vi "ReadDriverParameters.vi"(8 "error in (no error)":errorcluster) -> (0 "error out":errorcluster, 2 "DRV stand":T1)   [LabVIEW 2018, in "Application.lvlib"]
doc: "Read Driver Parameters in an Excel file"
uses:
  Application/Application.lvlib
  Application/DRV stand.ctl
  <vilib>/Utility/NIReport.llb/Report Type.ctl
  <vilib>/addons/_office/excel.llb/Excel Get Data ([str]).vi
  <vilib>/Utility/NIReport.llb/NI_report.lvclass
  <vilib>/Utility/NIReport.llb/Excel/NI_Excel.lvclass
  <vilib>/addons/_office/NI_ReportGenerationToolkit.lvlib
  <vilib>/Utility/NIReport.llb/NI_ReportGenerationCore.lvlib
panel:
  in  "effeciency":bool
  in  "DCI":bool
  in  "DCV":bool=TRUE
  in  "kW":bool=TRUE
  in  "PF":bool=TRUE
  in  "ACI":bool=TRUE
  in  "ACV":bool=TRUE
  in  "Cancel":bool
  out "Name":string
  out "effect min":dbl caption="HIÖU SUÊT"
  out "effect max":dbl caption="HIÖU SUÊT"
  out "DCI(mA) min":dbl caption="§IÖN ¸P DC (mA)"
  out "DCI(mA) max":dbl caption="§IÖN ¸P DC (mA)"
  out "DCV(Volts) min":dbl caption="§IÖN ¸P DC (Volts)"
  out "DCV(Volts) max":dbl caption="§IÖN ¸P DC (Volts)"
  out "AC kW (W) min":dbl caption="C¤NG SUÊT AC (Watt)"
  out "AC kW (W) max":dbl caption="C¤NG SUÊT AC (Watt)"
  out "pf min":dbl caption="HÖ Sè C¤NG SUÊT"
  out "pf  max":dbl caption="HÖ Sè C¤NG SUÊT"
  out "ACI(mA) min":dbl caption="DßNG §IÖN AC (mA)"
  out "ACI(mA) max":dbl caption="DßNG §IÖN AC (mA)"
  out "ACV(Volts) min":dbl caption="§iÖn ¸p AC (Volts)"
  out "ACV(Volts) max":dbl caption="§iÖn ¸p AC (Volts)"
  in  "Select Excel File":bool
  in  "Select":bool
  in  "ID":u16(ring) items=["00037845", "00032982", "00035647", "00035625", "00029051", "00039782", "00039558", "00041093", "00039479", "00022963", "00027236", "00029031", "00040386", "00040388", "00040390", "00030784", "00040761", "00040392", "00040394", "00040396", "00039185", "00041068", "00041072", "00041471", "00041079", "00027769", "00018946", "00026890", "00023932", "00040779", "00026346", "00027544", "00028946", "00039696", "00023152", "00015630", "00034834", "00035257", "00035244", "00041789", "00027814", "00028354", "00032423", "00031816", "00041407", "00039539", "00039236"]
  out "Parameters":string[](array[string])
  # "DRIVER"
  # "Parameters"
  # "MAX"
  # "MIN"
  # "§IÖN ¸P AC (Volts)"
  # "Dßng §IÖn AC (mA)"
  # "HÖ sè c«ng suÊt"
  # "c«ng suÊt AC (Watt)"
  # "§IÖN ¸P DC (VOLTS)"
  # "DßNG §IÖN DC (mA)"
  # "HIÖU SUÊT"
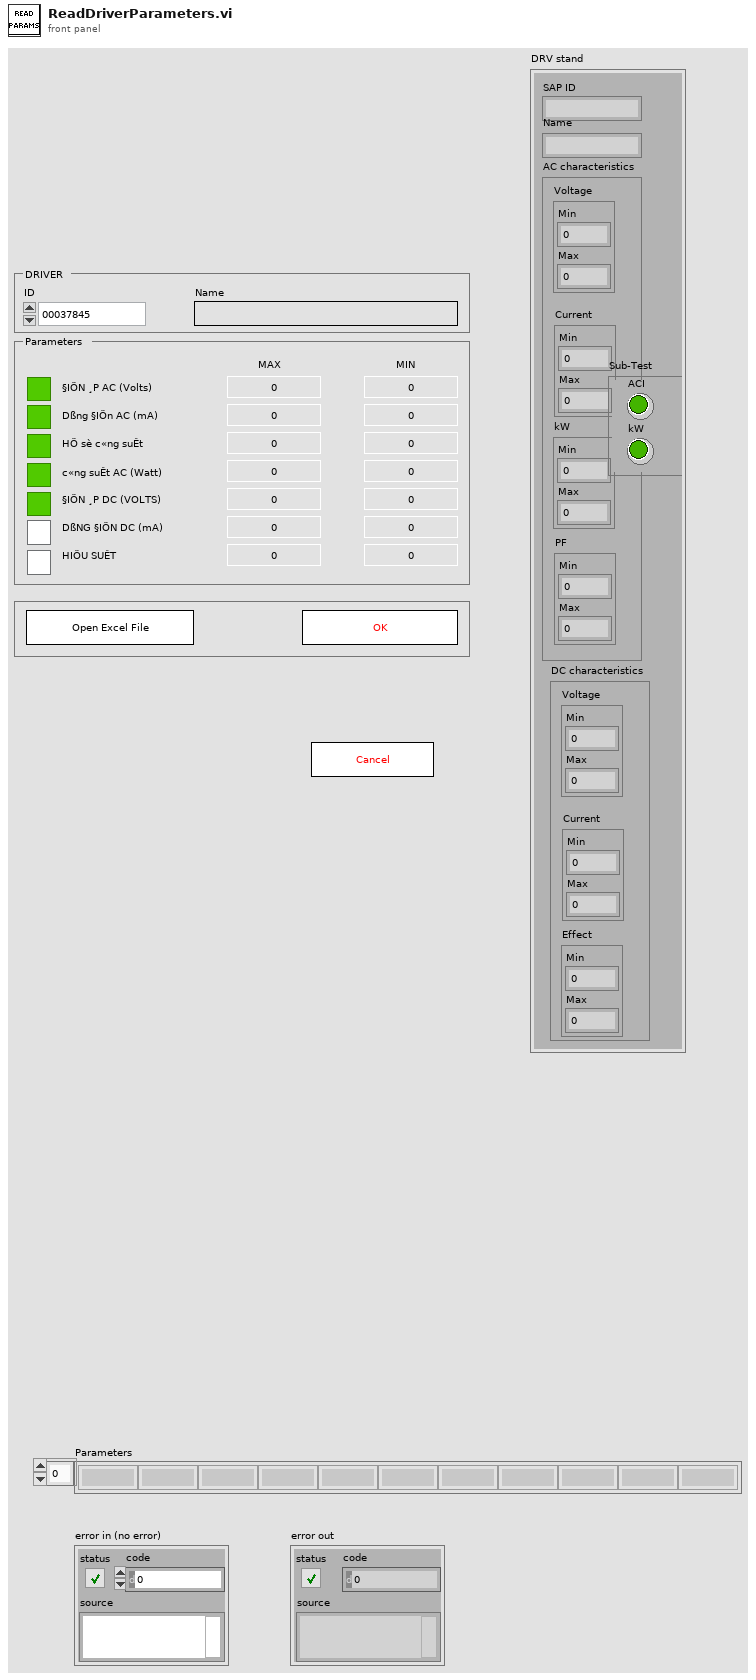
[diagram p1: front panel]
types:
  T1 = typedef "Application.lvlib/DRV stand.ctl" = cluster{"SAP ID":string, "Name":string, "AC characteristics":cluster{"Voltage":cluster{"Min":dbl, "Max":dbl}, "Current":cluster{"Min":dbl, "Max":dbl}, "kW":cluster{"Min":dbl, "Max":dbl}, "PF":cluster{"Min":dbl, "Max":dbl}}, "DC characteristics":cluster{"Voltage":cluster{"Min":dbl, "Max":dbl}, "Current":cluster{"Min":dbl, "Max":dbl}, "Effect":cluster{"Min":dbl, "Max":dbl}}, "Sub-Test":cluster{"ACV":bool, "ACI":bool, "kW":bool, "PF":bool, "DCV":bool, "DCI":bool, "efficiency":bool}}
  T2 = enum16{"maximized", "minimized", "normal", "no change"}
  T3 = typedef "NI_ReportGenerationCore.lvlib/Report Type.ctl" = enum16{"HTML", "Word", "Excel"}
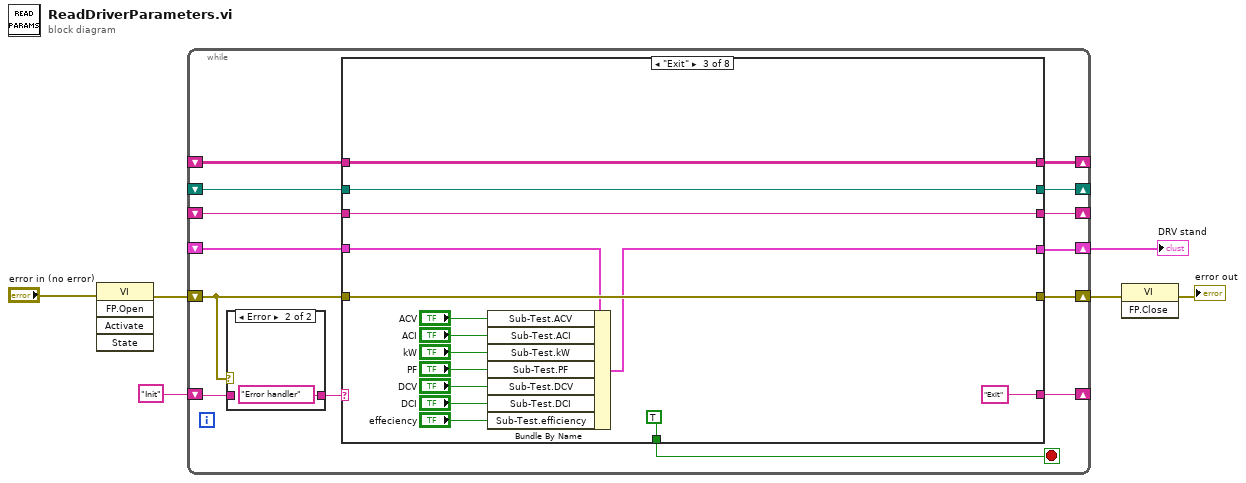
[diagram p0: block diagram]
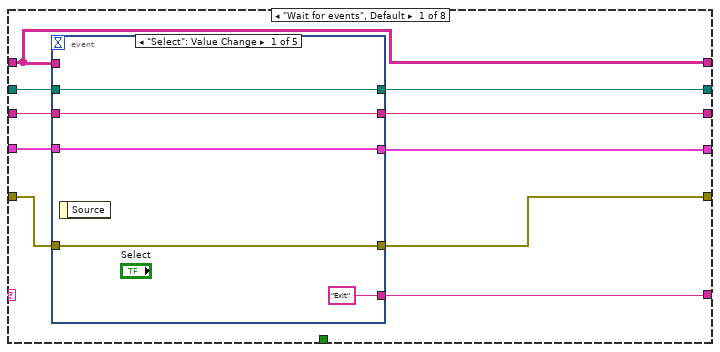
[diagram p3: hidden frame]
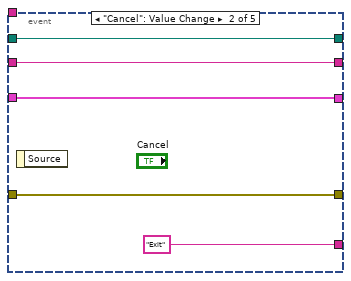
[diagram p4: hidden frame]
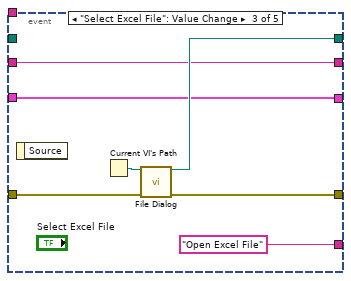
[diagram p5: hidden frame]
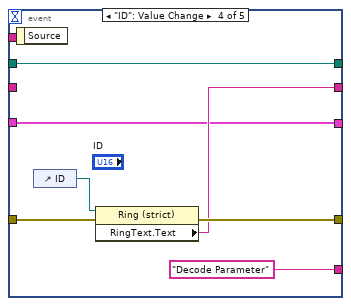
[diagram p6: hidden frame]
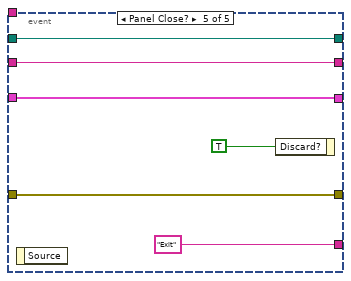
[diagram p7: hidden frame]
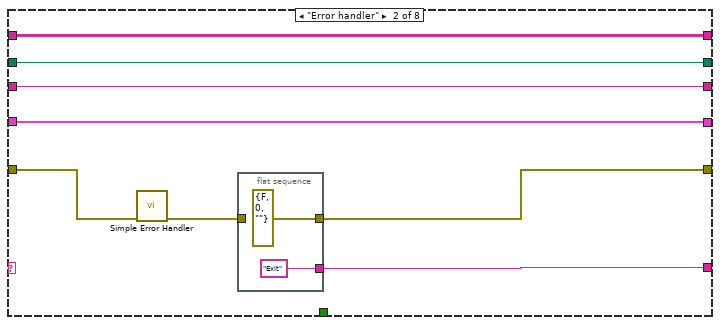
[diagram p8: hidden frame]
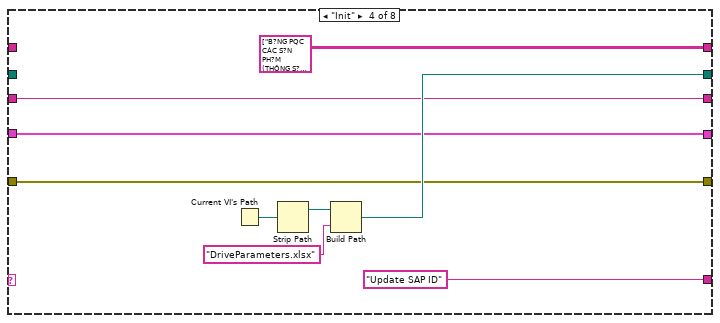
[diagram p9: hidden frame]
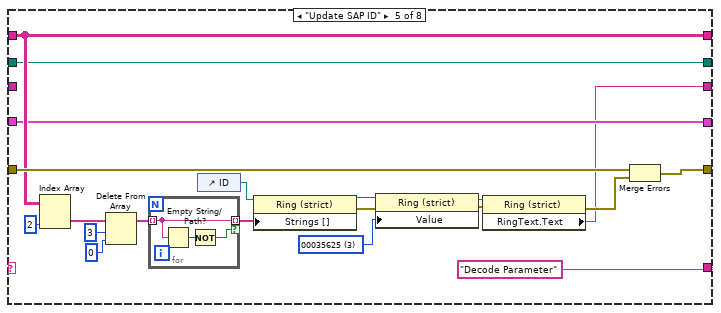
[diagram p10: hidden frame]
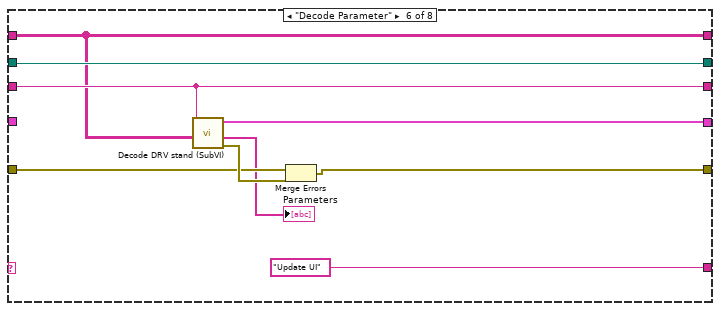
[diagram p11: hidden frame]
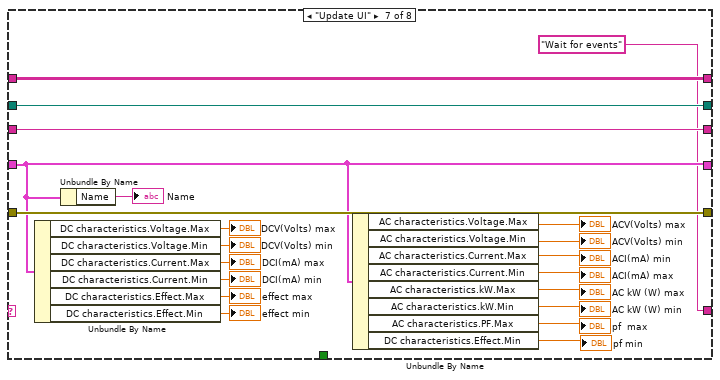
[diagram p12: hidden frame]
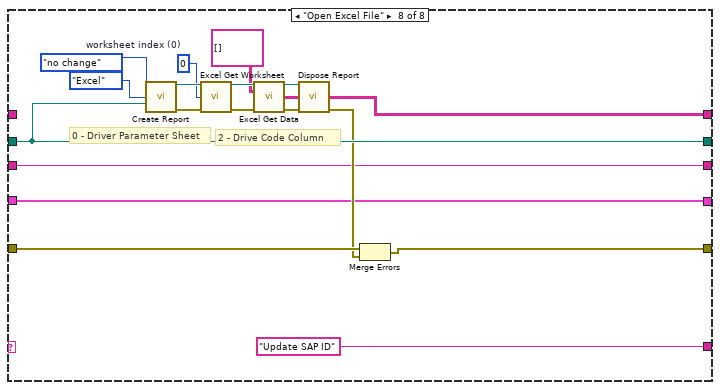
[diagram p13: hidden frame]
diagram:
  n1 = invoke class="VI" method="FP.Open"(error in="error in (no error)") -> (error out=w3:errorcluster)  [unwired: 4 in, 4 out]
  n2 = while {
    shift-right: [w20] -> _
    shift-left: "Init" -> [w17]
    shift-right: [w14] -> w6
    shift-left: w3 -> [w18]
    shift-right: [w15] -> _
    shift-left: _ -> [w11]
    shift-right: [w13] -> _
    shift-left: _ -> [w12]
    shift-right: [w7] -> w1
    shift-left: _ -> [w10]
    shift-right: [w9] -> _
    shift-left: _ -> [w8]
    stop <- w19 stop-if-true
    n3 = case shown="Error" w18 {
      tunnel: w17 -> [w21 _]
      tunnel: [w21 "Error handler"] -> w16
      frame No Error {
      }
      frame Error {
      }
    }
    n4 = case shown="\"Exit\"" w16 {
      tunnel: [_ _ TRUE _ _ _ _ _] -> w19
      tunnel: [w32 w69 "Exit" "Update SAP ID" "Decode Parameter" "Update UI" "Wait for events" "Update SAP ID"] -> w20
      tunnel: w18 -> [w30 w70 w83 w88 w116 w124 w148 w155]
      tunnel: [w31 w68 w85 w93 w108 w128 w149 w157] -> w15
      tunnel: [w29 w66 w83 w88 w107 w127 w148 w154] -> w14
      tunnel: [w27 w67 w84 string[][] [["B?NG PQC CÁC S?N PH?M (THÔNG S? QUANG ÐI?N)", "", "", "", "", "", "", "", "", "", "", "", "", ""], ["STT", "Tên s?n ph?m", "Mã SAP", "Ði?n áp (VAC)", "", "Dòng di?n vào AC", "Công suât (W)", "", "H? s? công su?t                    (PF)", "Ði?n áp trên module LED (VDC)", "", "Dòng ra ML LED\n(mA)", "", "Hi?u su?t di?n"], ["", "", "", "Min", "Max", "mA", "Min", "Max", "", "Min", "Max", "Min", "Max", "%"], ["1", "Driver Bulb A60 8W V1 TC", "00037845", "218", "222", "= 90", "7.2", "8.8", " = 0.45", "55", "65", "112", "123", " = 86"], ["2", "Driver TR100/20W.EV TC V1", "00032982", "218", "222", "= 250", "19", "22", " = 0.45", "", "", "", "", ""], ["3", "Driver BD M26 600/20W V1 TC", "00035647", "218", "222", "= 280", "18", "22", " = 0.45", "118", "142", "135", "155", " = 90"], ["4", "Driver BD M26 1200/40W V1 TC", "00035625", "218", "222", "= 550", "36", "44", " = 0.45", "118", "142", "270", "310", " = 90"], ["5", "Driver BD M36L 120/40W TC", "00029051", "218", "222", "= 450", "36", "44", " = 0.45", "118", "140", "280", "320", " = 92"], ["6", "B? Driver LED dây DR-LD01 60W(12VDC)", "00039782", "218", "222", "= 160", "11.5", "14.5", " = 0.45", "", "", "", "", ""], ["7", "Driver AT02-10 ÐM 9W IC BP2863SJ-TC", "00039558", "218", "222", "= 110", "7.6", "9.9", " = 0.45", "64", "76", "106", "118", " = 85"], ["8", "Driver AT10 ÐM 12W IC BP2863SJ(SS)-TC", "00041093", "218", "222", "= 160", "10.8", "13.2", " = 0.45", "81", "96", "118", "131", " = 85"], ["9", "Driver AT06L 5W IC BP2861BJ-TC", "00039479", "218", "222", "= 65", "4.2", "5.5", " = 0.45", "47", "58", "80", "90", " = 90"], ["10", "Driver Downlight 15W KC-TC", "00022963", "218", "222", "= 200", "14.4", "17.6", " = 0.45", "67", "79", "190", "210", " = 90"], ["11", "Driver D AT04L 155/16W -TC- Gi?c (EPC13)", "00027236", "218", "222", "= 200", "14.4", "17.6", " = 0.45", "67", "79", "190", "210", " = 90"], ["12", "Driver AT04L 7W-9W DE-TC", "00029031", "218", "222", "= 90", "6", "7.7", " = 0.45", "40", "50", "132", "146", " = 85"], ["13", "Driver AT04-10 7W IC BP2863SJ(DE)-TC", "00040386", "218", "222", "= 90", "6.4", "7.7", " = 0.45", "55", "65", "101", "112", " = 85"], ["14", "Driver AT04-10 9W IC BP2863SJ(DE)-TC", "00040388", "218", "222", "= 110", "8.3", "9.9", " = 0.45", "73", "85", "97", "108", " = 85"], ["15", "Driver AT04 12W IC BP2863SJ(DE)-TC", "00040390", "218", "222", "= 160", "10.8", "13.2", " = 0.45", "97", "114", "97", "108", " = 85"], ["16", "Driver AT06L 7W-9W DE-TC", "00030784", "218", "222", "= 90", "6", "7.7", " = 0.45", "40", "50", "132", "146", " = 85"], ["17", "Driver AT10L CCT - 7W - DE V2-TC", "00040761", "218", "222", "= 90", "6.4", "7.7", " = 0.45", "55", "65", "101", "112", " = 85"], ["18", "Driver AT02-10 ÐM 7W IC BP2863SJ(DE)-TC", "00040392", "218", "222", "= 90", "6.4", "7.7", " = 0.45", "55", "65", "101", "112", " = 85"], ["19", "Driver AT02-10 ÐM 9W IC BP2863SJ(DE)-TC", "00040394", "218", "222", "= 110", "8.3", "9.9", " = 0.45", "73", "85", "97", "108", " = 85"], ["20", "Driver AT10 ÐM 12W IC BP2863SJ(DE)-TC", "00040396", "218", "222", "= 160", "10.8", "13.2", " = 0.45", "97", "114", "97", "108", " = 85"], ["21", "Driver panel 7W-DE-TC", "00039185", "218", "222", "= 90", "6", "7.7", " = 0.45", "85", "95", "61", "68", " = 85"], ["22", "Driver panel 7W-DE V2-TC", "00041068", "218", "222", "= 90", "6", "7.7", " = 0.45", "85", "95", "61", "68", " = 85"], ["23", "Driver panel 12W-DE V2-TC", "00041072", "218", "222", "= 160", "10.8", "13.2", " = 0.45", "84", "99", "114", "126", " = 85"], ["24", "Driver panel CCT 9W-DE-TC", "00041471", "218", "222", "= 120", "7.4", "9.9", " = 0.45", "126", "148", "51", "57", " = 85"], ["25", "Driver panel CCT 12W-DE V2-TC", "00041079", "218", "222", "= 160", "10.5", "12.5", " = 0.45", "74.5", "78", "126", "140", " = 85"], ["26", "Driver PNL 320x1280-40W V1 KC TC", "00027769", "218", "222", "= 300", "38", "42", " = 0.9", "30", "42", "988", "1092", ""], ["27", "Driver PNL 320x1280-50W V1 KC RD", "00018946", "218", "222", "= 350", "45.5", "49", " = 0.9", "43.5", "45", "890", "490", ""], ["28", "Driver PNL 320x1280-50W CCT V1 KC TC", "00026890", "218", "222", "= 350", "45.5", "49", " = 0.9", "43.5", "45", "890", "490", ""], ["29", "Driver CSD05L/30W TC V1", "00023932", "218", "222", "= 250", "28", "33", " = 0.45", "105", "125", "223", "247", " = 90"], ["30", "Driver LED CSD02 40W (36W-V2 SC)", "00040779", "218", "222", "= 450", "36", "44", " = 0.95", "31.8", "37.5", "964", "1066", ""], ["31", "Driver D HB02L 350/50W (V4-Buck) TC", "00026346", "218", "222", "= 600", "42.5", "55", " = 0.9", "30", "40", "1140", "1260", " = 80"], ["32", "Driver D HB03L 290/100W (V1-Boost) TC", "00027544", "218", "222", "= 650", "96", "108", " = 0.9", "396", "446", "220", "244", ""], ["33", "Driver D HB03L 350/150W (V1-Boost-CTDA) TC", "00028946", "218", "222", "= 1100", "138", "162", " = 0.9", "396", "446", "327", "361", ""], ["34", "Driver CSC 200W TAU CA (LLC) V1 TC", "00039696", "218", "222", "850-900", "190", "200", " = 0.9", "100", "104", "1700", "1750", " = 90"], ["35", "Driver D CP06L/100W V5 TC", "00023152", "218", "222", "= 650", "96", "108", " = 0.9", "396", "446", "220", "244", ""], ["36", "Driver RL15-16-19 V2 TC", "00015630", "218", "222", "= 50", "4", "5.5", " = 0.45", "28", "34", "114", "126", ""], ["37", "Driver ÐB 6W RL36 DIM+CCT-TC (PCB tích h?p)", "00034834", "218", "222", "= 80", "5.4", "6.6", " = 0.45", "44", "54", "100", "110", " = 78"], ["38", "Driver dèn ch? I 30W-V2 TC (580MM)", "00035257", "219", "221", "172.5-287.5", "20.5", "24.5", " = 0.5", "150", "170", "123.5", "136.5", " = 90"], ["39", "Driver dèn ch? X 50W-V2 TC (580MM)", "00035244", "219", "221", "270-360", "37.5", "44", " = 0.5", "180", "200", "180.5", "199.5", " = 90"], ["40", "Driver TRL06 20W V1 TC", "00041789", "218", "222", "= 260", "18", "22", " = 0.5", "60", "72", "252", "278", " = 85"], ["41", "Driver Downlight 90/7W LPF DIM CCT RF V1 TC", "00027814", "218", "222", "= 120", "6", "8", " = 0.45", "28", "33", "180", "200", " = 78"], ["42", "Driver Downlight 110/9W LPF DIM CCT RF V1 TC", "00028354", "218", "222", "= 150", "8", "10", " = 0.45", "33", "40", "190", "210", " = 80"], ["43", "Driver D PT04L ÐM 12W.BLE-TC", "00032423", "218", "222", "= 220", "10.8", "13.2", " = 0.45", "70", "86", "", "135", " = 80"], ["44", "Driver P07 PANEL 40W.BLE V1 (DIM - CCT ) TC", "00031816", "218", "222", "= 400", "36", "45", " = 0.9", "32", "40", "902", "998", " = 80"], ["45", "Driver A60.PIR 9W V1 TC", "00041407", "218", "222", "= 90", "8.1", "9.9", " = 0.5", "", "", "", "", ""], ["46", "Driver OC.01.WF V1 - TC", "00039539", "218", "222", "= 15", "", "1", "", "", "", "", "", ""], ["47", "Driver dèn guong c?m bi?n G04.PIR 8W V2-TC", "00039236", "218", "222", "= 105", "7.1", "8.8", " = 0.5", "", "", "", "", ""], ["", "", "", "", "", "", "", "", "", "", "", "", "", ""], ["", "", "", "", "", "", "", "", "", "", "", "", "", ""], ["", "", "", "", "", "", "", "", "", "", "", "", "", ""], ["A", "Ghi chú: Ngành ÐTTÐ ch?t v?i Ban HT CNTT (H?o + Phú) theo b?ng này phù h?p th?c t? HT ngành dang áp d?ng  & H? th?ng  xu?ng. (Sheet 1. Scada TSQD (ch?t 22.7.21))", "", "", "", "", "", "", "", "", "", "", "", ""], ["Scada/ DASH BOARD", "1. Tên s?n ph?m nh?p kho + mã SAP d?ng b? theo KHSX d?n khâu nh?p kho t? LR Drv LED (theo tên s?n ph?m)", "", "", "", "", "", "", "", "", "", "", "", ""], ["", "2. Thông s? do 100% quá trình SX, nh?p theo PQC tên s?n ph?m b?ng trên, báo cáo A Kiên xây d?ng ph?n m?m scada dua lên Dashboard.", "", "", "", "", "", "", "", "", "", "", "", ""], ["", "3. Các SPM c?p nh?t b? sung  (KTV công ngh? ch?t lu?ng nh?p),  g?i l?i  Anh Kiên làm ph?n m?m nh?p b? sung khi phát sinh.", "", "", "", "", "", "", "", "", "", "", "", ""], ["", "4. Thông tin ngo?i quan ki?m soát quá trình: (sheet 2. Ngo?i quan (ch?t 14_7_21) Anh Kiên dua lên Dashboard.", "", "", "", "", "", "", "", "", "", "", "", ""], ["", "", "", "", "", "", "", "", "", "", "", "", "", ""], ["B", "1. KTV làm HDCV theo công do?n LR DRV LED ghép theo t?ng bu?c vi?c hi?n t?i (dã làm)", "", "", "", "", "", "", "", "", "", "", "", ""], ["HDCV", "2. Tên HDCV theo tên dòng SP/ ch?ng lo?i/ công su?t (nhu dang làm trên Online)", "", "", "", "", "", "", "", "", "", "", "", ""], ["", "3. KTV + TPCL g?i trên WEB  v?: http://192.168.68.88/custom/document-list/.., nhu dang xem online và in ra hàng ngày (Mr Phú hu?ng d?n cách ghép màn hình t? 24/7/2021)", "", "", "", "", "", "", "", "", "", "", "", ""], ["", "(riêng HDCV d?t tên theo Format c?a HT Online dang có)", "", "", "", "", "", "", "", "", "", "", "", ""], ["", "", "", "", "", "", "", "", "", "", "", "", "", ""], ["", "", "", "", "", "", "", "", "", "", "", "", "", ""], ["", "", "", "", "", "", "", "", "", "", "", "", "", ""], ["", "", "", "", "", "", "", "", "", "", "", "", "", ""], ["", "", "", "", "", "", "", "", "", "", "", "", "", ""], ["", "", "", "", "", "", "", "", "", "", "", "", "", ""], ["", "", "", "", "", "", "", "", "", "", "", "", "", ""], ["", "", "", "", "", "", "", "", "", "", "", "", "", ""], ["", "", "", "", "", "", "", "", "", "", "", "", "", ""], ["", "", "", "", "", "", "", "", "", "", "", "", "", ""], ["", "", "", "", "", "", "", "", "", "", "", "", "", ""], ["", "", "", "", "", "", "", "", "", "", "", "", "", ""], ["", "", "", "", "", "", "", "", "", "", "", "", "", ""], ["", "", "", "", "", "", "", "", "", "", "", "", "", ""], ["", "", "", "", "", "", "", "", "", "", "", "", "", ""], ["", "", "", "", "", "", "", "", "", "", "", "", "", ""], ["", "", "", "", "", "", "", "", "", "", "", "", "", ""], ["", "", "", "", "", "", "", "", "", "", "", "", "", ""], ["", "", "", "", "", "", "", "", "", "", "", "", "", ""], ["", "", "", "", "", "", "", "", "", "", "", "", "", ""], ["", "", "", "", "", "", "", "", "Hà N?i, ngày 22 tháng 7 nam 2021", "", "", "", "", ""], ["", "", "", "", "", "", "", "", "Ngành ÐTTÐ", "", "", "", "", ""]] ("contents") w109 w120 w147 w156] -> w13
      tunnel: w12 -> [w27 w67 w84 _ w109 w120 w147 _]
      tunnel: w11 -> [w28 w68 w85 _ w108 w128 w149 w157]
      tunnel: [w26 w65 w75 w90 w106 w121 w138 w152] -> w7
      tunnel: w10 -> [w25 w65 w74 w90 w106 _ w138 w152]
      tunnel: [w24 w64 w82 w89 w102 w125 w146 w151] -> w9
      tunnel: w8 -> [w23 w64 w82 w89 _ w125 w146 w151]
      frame "Wait for events", Default {
        n5 = event shown="[0] \"Select\": Value Change" {
          selector: _ -> [_ _ _ _ _]
          dyn-events: _ -> [_ _ _ _ _]
          timeout: _ -> [_ _ _ _ _]
          tunnel: ["Exit" "Exit" "Open Excel File" "Decode Parameter" "Exit"] -> w32
          tunnel: [w36 w41 w49 w50 w57] -> w31
          tunnel: w30 -> [w35 w40 w46 w55 w59]
          tunnel: [w35 w40 w45 w54 w59] -> w29
          tunnel: w28 -> [w36 w41 _ w50 w57]
          tunnel: w27 -> [_ _ _ _ _]
          tunnel: [w34 w39 w44 w51 w60] -> w26
          tunnel: w25 -> [w34 w39 w44 w51 w60]
          tunnel: [w33 w38 w43 w52 w58] -> w24
          tunnel: w23 -> [w33 w38 w43 _ w58]
          event "Select": Value Change {
            n6 = event-data() -> ()  [unwired: 1 in, 1 out]
          }
          event "Cancel": Value Change {
            n7 = event-data() -> ()  [unwired: 1 in, 1 out]
          }
          event "Select Excel File": Value Change {
            n8 = event-data() -> ()  [unwired: 1 in, 1 out]
            n9 = Current VI's Path() -> (path=w48:path)
            n10 = call "File Dialog"("start path"=w48, "error in"=w46) -> ("selected path"=w49:path, "error out"=w45:errorcluster)  [unwired: 10 in, 2 out]
          }
          event "ID": Value Change {
            n11 = event-data() -> ()  [unwired: 1 in, 1 out]
            n12 = control-ref of="ID"() -> (w56:refnum<vi>)
            n13 = property class="Ring (strict)"(reference=w56, error in=w55) -> (error out=w54:errorcluster, "RingText.Text"=w52:string)  [unwired: 1 out]
          }
          event Panel Close? {
            n14 = event-data() -> ()  [unwired: 1 in, 1 out]
            n15 = event-data("Discard?"=TRUE) -> ()  [unwired: 1 in, 1 out]
          }
        }
      }
      frame "Error handler" {
        n16 = call <vilib>:"Simple Error Handler.vi"("error in (no error)"=w70) -> ("error out"=w63:errorcluster)  [unwired: 1 in, 7 out]
        n17 = flat-sequence {
          tunnel: ["Exit"] -> w69
          tunnel: [errorcluster {"status"=FALSE, "code"=0, "source"=""} ("error constant")] -> w66
          tunnel: w63 -> [_]
          frame #0 {
          }
        }
      }
      frame "Exit" {
        n18 = Bundle By Name(cluster=w74, "Sub-Test.ACV"="ACV", "Sub-Test.ACI"="ACI", "Sub-Test.kW"="kW", "Sub-Test.PF"="PF", "Sub-Test.DCV"="DCV", "Sub-Test.DCI"="DCI", "Sub-Test.efficiency"="effeciency") -> (w75:T1)
      }
      frame "Init" {
        n19 = Current VI's Path() -> (path=w95:path)
        n20 = Strip Path(path=w95) -> (stripped path=w96:path)  [unwired: 1 out]
        n21 = Build Path(base path=w96, name or relative path="DriveParameters.xlsx") -> (appended path=w93:path)
      }
      frame "Update SAP ID" {
        w97 = u16 3 items=["00037845", "00032982", "00035647", "00035625", "00029051", "00039782", "00039558", "00041093", "00039479", "00022963", "00027236", "00029031", "00040386", "00040388", "00040390", "00030784", "00040761", "00040392", "00040394", "00040396", "00039185", "00041068", "00041072", "00041471", "00041079", "00027769", "00018946", "00026890", "00023932", "00040779", "00026346", "00027544", "00028946", "00039696", "00023152", "00015630", "00034834", "00035257", "00035244", "00041789", "00027814", "00028354", "00032423", "00031816", "00041407", "00039539", "00039236"] ("ID")
        n22 = Index Array(array=w109, index (col)=2 ("disabled index (col)")) -> (element=w115:string[])  [unwired: 1 in]
        n23 = Delete From Array(array=w115, length=3, index=0) -> (array with subset deleted=w112:string[])  [unwired: 1 out]
        n24 = for {
          tunnel: w112 -> [w118] mode=indexing
          tunnel: [w118] -> w111 mode=indexing if=w117
          n25 = Empty String/Path?(string/path=w118) -> (empty?=w119:bool)
          n26 = Not(x=w119) -> (.not. x?=w117:bool)
        }
        n27 = control-ref of="ID"() -> (w110:refnum<vi>)
        n28 = property class="Ring (strict)"(reference=w110, "Strings []"=w111) -> (reference out=w100:refnum<vi>, error out=w101:errorcluster)  [unwired: 1 in]
        n29 = property class="Ring (strict)"(reference=w100, error in=w101, "Value"=w97) -> (reference out=w98:refnum<vi>, error out=w99:errorcluster)
        n30 = property class="Ring (strict)"(reference=w98, error in=w99) -> (error out=w103:errorcluster, "RingText.Text"=w102:string)  [unwired: 1 out]
        n31 = Merge Errors(w116, w103) -> (w107:errorcluster)
      }
      frame "Decode Parameter" {
        n32 = call "Decode DRV stand (SubVI).vi"("Excel Data"=w120, "SAP ID"=w125) -> ("error out"=w126:errorcluster, "subarray"=→"Parameters":string[], "DRV stand"=w121:T1)  [unwired: 7 in]
        n33 = Merge Errors(w124, w126) -> (w127:errorcluster)
      }
      frame "Update UI" {
        n34 = Unbundle By Name(w138) -> ("DC characteristics.Voltage.Max"=→"DCV(Volts) max":dbl, "DC characteristics.Voltage.Min"=→"DCV(Volts) min":dbl, "DC characteristics.Current.Max"=→"DCI(mA) max":dbl, "DC characteristics.Current.Min"=→"DCI(mA) min":dbl, "DC characteristics.Effect.Max"=→"effect max":dbl, "DC characteristics.Effect.Min"=→"effect min":dbl)
        n35 = Unbundle By Name(w138) -> ("Name"=→"Name":string)
        n36 = Unbundle By Name(w138) -> ("AC characteristics.Voltage.Max"=→"ACV(Volts) max":dbl, "AC characteristics.Voltage.Min"=→"ACV(Volts) min":dbl, "AC characteristics.Current.Max"=→"ACI(mA) min":dbl, "AC characteristics.Current.Min"=→"ACI(mA) max":dbl, "AC characteristics.kW.Max"=→"AC kW (W) max":dbl, "AC characteristics.kW.Min"=→"AC kW (W) min":dbl, "AC characteristics.PF.Max"=→"pf  max":dbl, "DC characteristics.Effect.Min"=→"pf min":dbl)
      }
      frame "Open Excel File" {
        w158 = 0  # worksheet index (0)
        # "0 - Driver Parameter Sheet"
        # "2 - Drive Code Column"
        n37 = call <vilib>:"Create Report.vi"("window state (normal)"=T2."no change", "report type"=Report_Type."Excel", "template (empty)"=w157) -> ("report out"=w163:refnum<class "NI_report.lvclass">, "error out"=w162:errorcluster)  [unwired: 11 in]
        n38 = call <vilib>:"Excel Get Worksheet.vi"("report in"=w163, "worksheet index (0)"=w158, "error in (no error)"=w162) -> ("report out"=w164:refnum<class "NI_report.lvclass">, "error out"=w165:errorcluster)  [unwired: 11 out]
        n39 = call-poly <vilib>:"Excel Get Data.vi"("report in"=w164, "data type"=string[][] [], "error in (no error)"=w165) -> ("report out"=w166:refnum<class "NI_report.lvclass">, "data"=w156:string[][], "error out"=w167:errorcluster)  [unwired: 2 in, 8 out]
        n40 = call-dynamic "Dispose Report.vi"("report in"=w166, "error in (no error)"=w167) -> ("error out"=w153:errorcluster)  [unwired: 3 in, 10 out]
        n41 = Merge Errors(w155, w153) -> (w154:errorcluster)
      }
    }
  }
  "DRV stand" <- w1
  n42 = invoke class="VI" method="FP.Close"(error in=w6) -> (error out=→"error out":errorcluster)  [unwired: 2 in, 2 out]
